vi "Save to TDMS Core.vi"(8 "Error In":errorcluster, 10 "TDMS Ref":refnum<k34>, 11 "LHW-WfmData in":refnum<class "LHW-WfmData.lvclass">) -> (0 "Error Out":errorcluster, 3 "LHW-WfmData out":refnum<class "LHW-WfmData.lvclass">)   [LabVIEW 2016, in "LHW-Data.lvlib" / "LHW-WfmData.lvclass"]
doc: "Save data to TDMS file."
uses:
  LHW-WfmData.lvclass
  LHW-WfmData.lvclass/LHW-WfmData.ctl
  LHW-Data/LHW-Data.lvclass
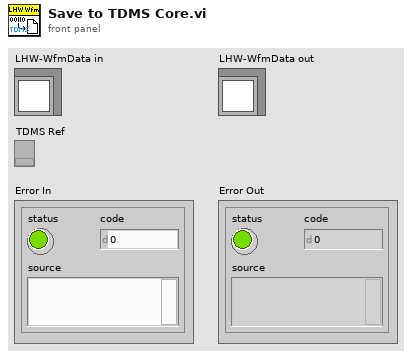
[diagram p1: front panel]
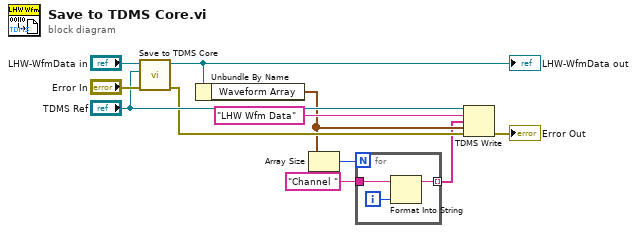
[diagram p0: block diagram]
diagram:
  n1 = call-parent "Save to TDMS Core.vi"("Error In"="Error In", "TDMS Ref"="TDMS Ref", "LHW-Data in"="LHW-WfmData in") -> ("Error Out"=w7:errorcluster, "LHW-Data out"=w9:refnum<class "LHW-WfmData.lvclass">)  [unwired: 7 in]
  "LHW-WfmData out" <- w9
  n2 = Unbundle By Name(w9) -> ("Waveform Array"=w4:waveform(dbl)[])
  n3 = Array Size(array=w4) -> (size(s)=w3:i32)
  n4 = for {
    N: w3 -> [_]
    tunnel: "Channel " ("group name in (Untitled)") -> [w14]
    tunnel: [w12] -> w1 mode=indexing
    i -> [w13]
    n5 = Format Into String(initial string=w14, w13) -> (resulting string=w12:string)  [unwired: 2 in, 1 out]
  }
  n6 = TDMS Write(0:"TDMS Ref", 5:"LHW Wfm Data" ("group name in (Untitled)"), 7:w1, 9:w4, 11:w7) -> (15:→"Error Out":errorcluster)  [unwired: 1 in, 3 out]
